vi "Configure Steering Frame.vi"(8 "error in (no error)":errorcluster, 10 "dialog options in":variant, 11 "steering frame in":refnum<class "NI_Robotics_Steering Frame.lvclass">) -> (0 "error out":errorcluster, 1 "cancelled?":bool, 2 "dialog options out":variant, 3 "steering frame out":refnum<class "NI_Robotics_Steering Frame.lvclass">, 5 "steering type":string)   [LabVIEW 2017, in "NI_Robotics_Configure Steering Frame.lvlib"]
uses:
  <vilib>/robotics/Dialog/Configure Steering Frame/NI_Robotics_Configure Steering Frame.lvlib
  <vilib>/robotics/Dialog/Configure Steering Frame/Steering Type.ctl
  <vilib>/robotics/Dialog/Configure Steering Frame/Zoom Extent.ctl
  <vilib>/robotics/Dialog/Configure Steering Frame/Zoom In.ctl
  <vilib>/robotics/Dialog/Configure Steering Frame/Zoom Out.ctl
  <vilib>/robotics/Dialog/Configure Steering Frame/Copy.ctl
  <vilib>/robotics/Dialog/Configure Steering Frame/Remove.ctl
  <vilib>/robotics/Dialog/Configure Steering Frame/Add.ctl
  <vilib>/robotics/Dialog/Configure Steering Frame/Angle Mode.ctl
  <vilib>/robotics/Steering/Steering Frame/NI_Robotics_Steering Frame.lvclass
  <vilib>/robotics/Dialog/Configure Steering Frame/FP Refs.ctl
  <vilib>/Utility/cursorutil.llb/Set Cursor (Icon Pict).vi
  <vilib>/robotics/Dialog/Configure Steering Frame/Global Strings.vi
panel:
  in  "Angle Units":T1=1 items=["Degrees", "Radians"]
  in  "help":bool
  in  "cancel":bool
  in  "ok":bool
  in  "Copy Wheel":T2
  in  "Remove Wheel":T3
  in  "Add Wheel":T4
  in  "Wheels":i32[](listbox)=[0]
  in  "zoom extent":T5 caption="Zoom to Fit"
  in  "zoom out":T6 caption="Zoom Out"
  in  "zoom in":T7 caption="Zoom In"
  in  "Steering Type":T8 items=["User Defined", "Differential", "Ackermann", "Mecanum"]
  out "picture":picture
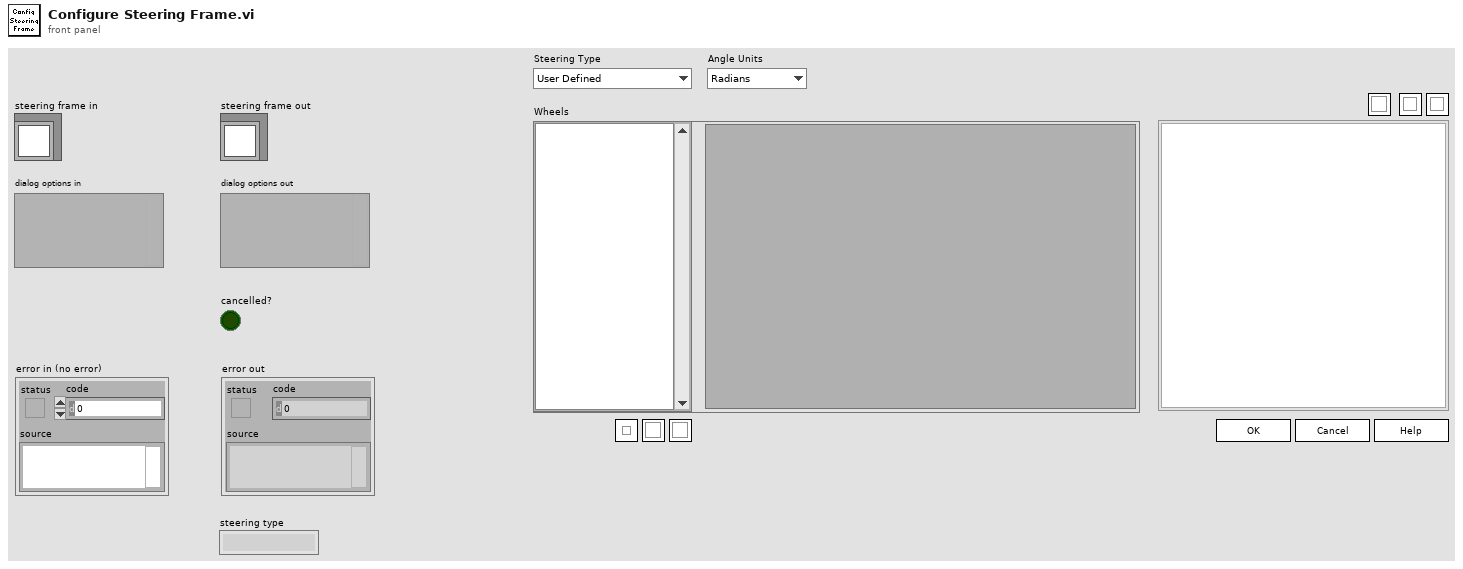
[diagram p1: front panel]
types:
  T1 = typedef "NI_Robotics_Configure Steering Frame.lvlib/Angle Mode.ctl" = u16
  T2 = typedef "NI_Robotics_Configure Steering Frame.lvlib/Copy.ctl" = bool
  T3 = typedef "NI_Robotics_Configure Steering Frame.lvlib/Remove.ctl" = bool
  T4 = typedef "NI_Robotics_Configure Steering Frame.lvlib/Add.ctl" = bool
  T5 = typedef "NI_Robotics_Configure Steering Frame.lvlib/Zoom Extent.ctl" = bool
  T6 = typedef "NI_Robotics_Configure Steering Frame.lvlib/Zoom Out.ctl" = bool
  T7 = typedef "NI_Robotics_Configure Steering Frame.lvlib/Zoom In.ctl" = bool
  T8 = typedef "NI_Robotics_Configure Steering Frame.lvlib/Steering Type.ctl" = u16
  T9 = typedef "NI_Robotics_Configure Steering Frame.lvlib/FP Refs.ctl" = cluster{"VI Refnum":refnum<vi>, "Menu Ref":refnum<k9>, "Sub Panel":refnum<vi>, "picture":refnum<vi>, "Steering Type":refnum<vi>, "zoom in":refnum<vi>, "zoom out":refnum<vi>, "zoom extents":refnum<vi>, "Wheels":refnum<vi>, "Add Wheel":refnum<vi>, "Remove Wheel":refnum<vi>, "Copy Wheel":refnum<vi>, "Angle Units":refnum<vi>}
  T10 = typedef "NI_Robotics_Configure Steering Frame.lvlib/Dialog Options.ctl" = cluster{"angle mode":T1, "picture pixels per unit":dbl, "close window on exit":bool, "window behavior":enum32{"Invalid", "Default", "Floating", "Floating/Auto-Hide", "Modal"}}
  T11 = typedef "NI_Robotics_Configure Steering Frame.lvlib/Subpanel to Main Command Event Reg.ctl" = refnum<event-registration>
  T12 = typedef "NI_Robotics_Configure Steering Frame.lvlib/Dialog Info.ctl" = cluster{"steering frame ref":refnum<data-value>, "active wheel indexes":i32[], "FP Refs":T9, "subpanel info":T13, "picture dragging state":T15, "picture size (pixels)":T17, "picture grid":picture, "click zones group":cluster{"click zones array":T18[], "num click zones":i32}, "draw options":T19}
  T13 = typedef "NI_Robotics_Configure Steering Frame.lvlib/Subpanel Info.ctl" = cluster{"subpanel VI refs":refnum<vi>[], "subpanel types":string[], "main to subpanel command events":T14[]}
  T14 = typedef "NI_Robotics_Configure Steering Frame.lvlib/Main to Subpanel Command Event.ctl" = refnum<user-event>
  T15 = typedef "NI_Robotics_Configure Steering Frame.lvlib/Dragging State.ctl" = cluster{"dragging":bool, "wheel index":i32, "dragging mode":T16, "wheel start position":cluster{"x":dbl, "y":dbl, "theta":dbl}, "relative mouse position":cluster{"x":dbl, "y":dbl}, "relative mouse init angle (rad)":dbl}
  T16 = typedef "NI_Robotics_Configure Steering Frame.lvlib/Dragging Mode.ctl" = enum16{"translate", "rotate"}
  T17 = typedef "LVBoundsTypeDef.ctl" = cluster{"Width":u32, "Height":u32}
  T18 = typedef "NI_Robotics_Configure Steering Frame.lvlib/Click Zone.ctl" = cluster{"wheel index":i32, "global coordinate":cluster{"x":dbl, "y":dbl}, "radius":dbl}
  T19 = typedef "NI_Robotics_Steering Picture.lvlib/Draw Steering Frame Options.ctl" = cluster{"draw wheel states?":bool, "highlight wheel index":i32, "pixels per unit":dbl, "draw forward velocity?":bool, "velocity scale":dbl}
  T20 = typedef "eventvkey.ctl" = enum16{"ASCII", "Enter", "Return", "Shift", "Ctrl", "Alt", "Cmd", "Opt", "Caps", "NumLock", "Clear", "Break", "Up", "Down", "Left", "Right", "Insert", "Delete", "Home", "End", "PageUp", "PageDown", "Escape", "Help", "Pause", "ScrollLock", "F1", "F2", "F3", "F4", "F5", "F6", "F7", "F8", "F9", "F10", "F11", "F12", "F13", "F14", "F15", "F16", "F17", "F18", "F19", "F20", "F21", "F22", "F23", "F24", "Play", "VolumeUp", "VolumeDown", "Mute", "Two Byte Char"}
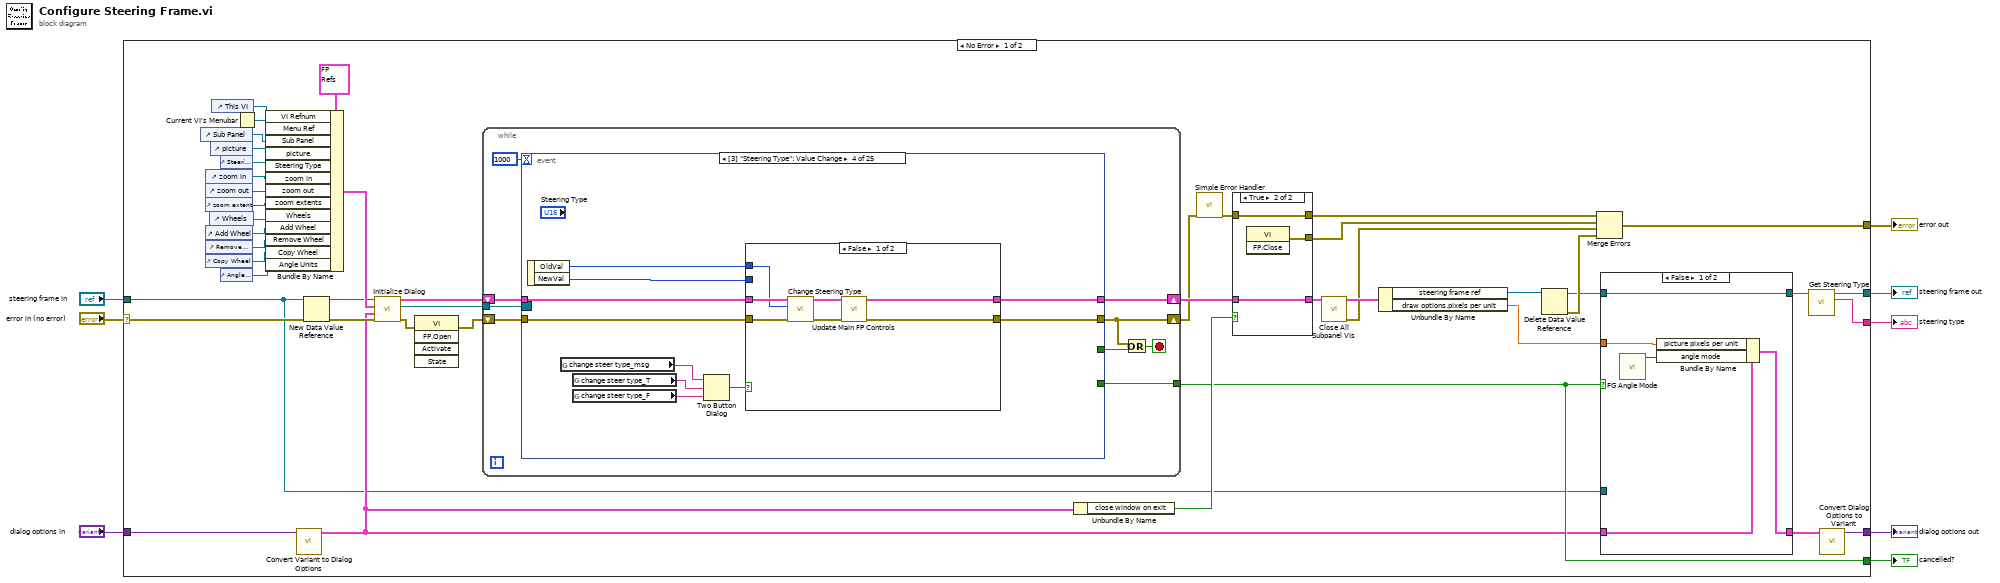
[diagram p0: block diagram]
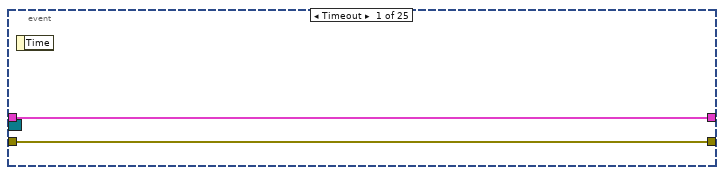
[diagram p4: hidden frame]
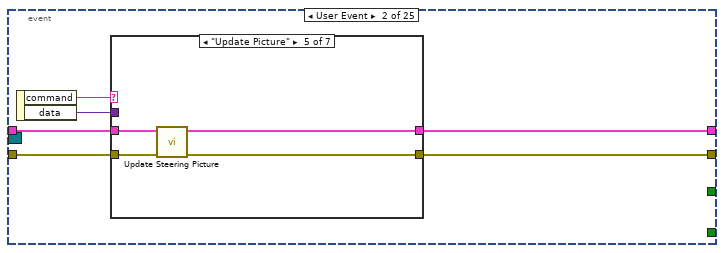
[diagram p5: hidden frame]
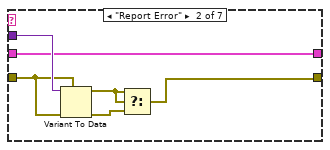
[diagram p7: hidden frame]
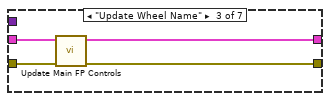
[diagram p8: hidden frame]
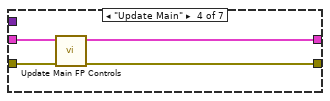
[diagram p9: hidden frame]
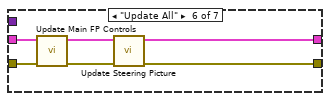
[diagram p10: hidden frame]
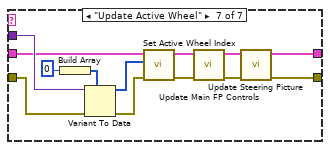
[diagram p11: hidden frame]
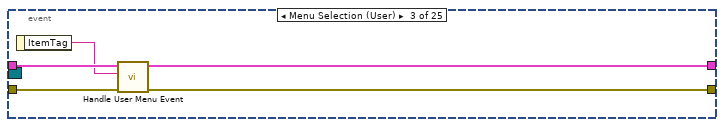
[diagram p12: hidden frame]
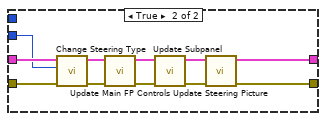
[diagram p13: hidden frame]
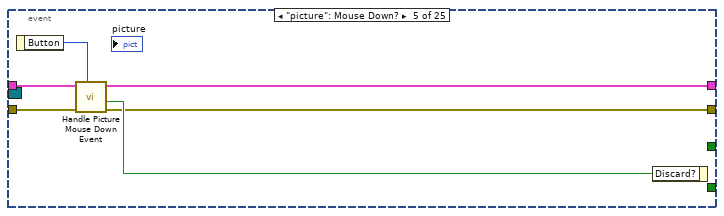
[diagram p14: hidden frame]
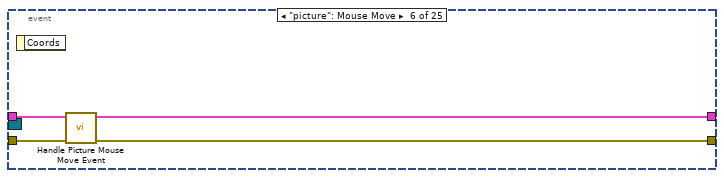
[diagram p15: hidden frame]
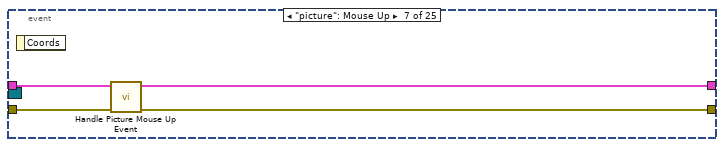
[diagram p16: hidden frame]
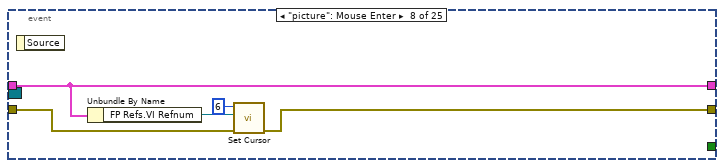
[diagram p17: hidden frame]
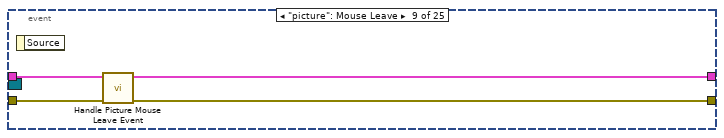
[diagram p18: hidden frame]
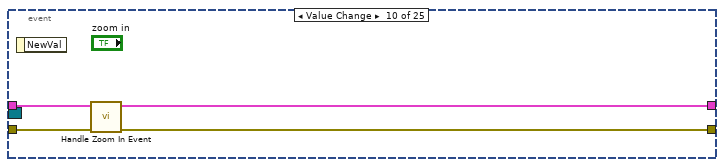
[diagram p19: hidden frame]
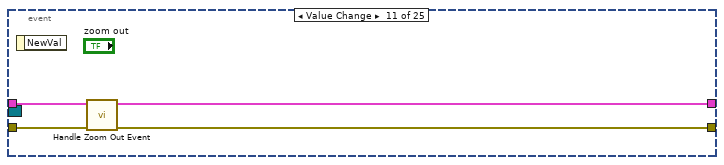
[diagram p20: hidden frame]
diagram:
  n1 = case shown="No Error" "error in (no error)" {
    selector: "error in (no error)" -> [w25 w319]
    tunnel: [w15 w317] -> w1
    tunnel: [w32 _] -> w8
    tunnel: "dialog options in" -> [w21 w318]
    tunnel: [w19 w318] -> w6
    tunnel: [w30 w319] -> w3
    tunnel: [w16 _] -> w4
    tunnel: "steering frame in" -> [w9 w317]
    frame No Error {
      n2 = control-ref of="Sub Panel"() -> (w52:refnum<vi>)
      n3 = control-ref of="zoom in"() -> (w29:refnum<vi>)
      n4 = control-ref of="zoom out"() -> (w28:refnum<vi>)
      n5 = control-ref of="zoom extent"() -> (w27:refnum<vi>)
      n6 = control-ref of="Add Wheel"() -> (w24:refnum<vi>)
      n7 = control-ref of="Remove Wheel"() -> (w23:refnum<vi>)
      n8 = control-ref of="Copy Wheel"() -> (w22:refnum<vi>)
      n9 = control-ref of="Wheels"() -> (w14:refnum<vi>)
      n10 = control-ref of="picture"() -> (w48:refnum<vi>)
      n11 = control-ref of="This VI"() -> (w46:refnum<vi>)
      n12 = control-ref of="Steering Type"() -> (w11:refnum<vi>)
      n13 = control-ref of="Angle Units"() -> (w10:refnum<vi>)
      n14 = Current VI's Menubar() -> (w31:refnum<k9>)
      n15 = Bundle By Name(cluster=T9 {"VI Refnum"=refnum, "Menu Ref"=refnum, "Sub Panel"=refnum, "picture"=refnum, "Steering Type"=refnum, "zoom in"=refnum, "zoom out"=refnum, "zoom extents"=refnum, "Wheels"=refnum, "Add Wheel"=refnum, "Remove Wheel"=refnum, "Copy Wheel"=refnum, "Angle Units"=refnum} ("FP Refs"), "VI Refnum"=w46, "Menu Ref"=w31, "Sub Panel"=w52, "picture"=w48, "Steering Type"=w11, "zoom in"=w29, "zoom out"=w28, "zoom extents"=w27, "Wheels"=w14, "Add Wheel"=w24, "Remove Wheel"=w23, "Copy Wheel"=w22, "Angle Units"=w10) -> (w49:T9)
      n16 = call <vilib>:"Convert Variant to Dialog Options.vi"("dialog options variant"=w21) -> ("dialog options"=w20:T10)  [unwired: 9 in, 1 out]
      n17 = New Data Value Reference(data value=w9, error in=w25) -> (data value reference=w43:refnum<data-value>, error out=w42:errorcluster)
      n18 = call <vilib>:"Initialize Dialog.vi"("error in (no error)"=w42, "dialog options in"=w20, "FP Refs"=w49, "steering frame ref in"=w43) -> ("error out"=w45:errorcluster, "subpanel to main command event reg"=w51:T11, "dialog info"=w50:T12)  [unwired: 5 in]
      n19 = invoke class="VI" method="FP.Open"(error in=w45) -> (error out=w44:errorcluster)  [unwired: 4 in, 4 out]
      n20 = while {
        shift-right: [w66] -> w13
        shift-left: w44 -> [w73]
        tunnel: w51 -> [w74]
        shift-right: [w68] -> w40
        shift-left: w50 -> [w71]
        tunnel: [w67] -> w32
        stop <- w70 stop-if-true
        n21 = event shown="[3] \"Steering Type\": Value Change" {
          selector: w74 -> [_ _ _ _ _ _ _ _ _ _ _ _ _ _ _ _ _ _ _ _ _ _ _ _ _]
          dyn-events: _ -> [_ _ _ _ _ _ _ _ _ _ _ _ _ _ _ _ _ _ _ _ _ _ _ _ _]
          timeout: 1000 -> [_ _ _ _ _ _ _ _ _ _ _ _ _ _ _ _ _ _ _ _ _ _ _ _ _]
          tunnel: w73 -> [w76 w80 w124 w135 w156 w163 w166 w170 w175 w179 w183 w190 w194 w198 w207 w231 w236 w241 w266 w282 w296 w300 w304 w306 w316]
          tunnel: [w76 w79 w123 w134 w158 w161 w165 w169 w174 w178 w182 w187 w193 w202 w206 w230 w235 w248 w262 w278 w290 w300 w304 w305 w316] -> w66
          tunnel: [w75 w77 w125 w132 w159 w162 w167 w171 w176 w180 w184 w188 w195 w204 w208 w232 w237 w249 w263 w279 w293 w301 w303 w309 w315] -> w68
          tunnel: w71 -> [w75 w78 w126 w133 w157 w164 w168 w171 w177 w181 w185 w189 w196 w201 w209 w233 w238 w243 w267 w283 w294 w301 w303 w309 w315]
          tunnel: [_ _ _ _ _ _ _ _ _ _ _ _ _ _ _ _ _ _ _ _ _ TRUE w302 _ w310] -> w69
          tunnel: [_ _ _ _ _ _ _ _ _ _ _ _ _ _ _ _ _ _ _ _ _ _ w302 _ w310] -> w67
          event Timeout {
            n22 = event-data() -> ()  [unwired: 1 in, 1 out]
          }
          event User Event {
            n23 = event-data() -> ("command"=w82:string, "data"=w81:variant)  [unwired: 1 in]
            n24 = case shown="\"Update Picture\"" w82 {
              tunnel: w81 -> [_ w90 _ _ _ _ w121]
              tunnel: w80 -> [w84 w89 w92 w96 w101 w107 w120]
              tunnel: [w84 w86 w91 w95 w99 w103 w116] -> w79
              tunnel: w78 -> [w83 w85 w94 w98 w102 w108 w115]
              tunnel: [w83 w85 w93 w97 w100 w104 w117] -> w77
              frame Default {
              }
              frame "Report Error" {
                n25 = Variant To Data(error in=w89, type=w89, Variant=w90) -> (data=w88:errorcluster, error out=w87:errorcluster)
                n26 = Select(t=w88, s=w88, f=w87) -> (s? t:f=w86:errorcluster)
              }
              frame "Update Wheel Name" {
                n27 = call <vilib>:"Update Main FP Controls.vi"("error in (no error)"=w92, "dialog info in"=w94) -> ("error out"=w91:errorcluster, "dialog info out"=w93:T12)  [unwired: 8 in]
              }
              frame "Update Main" {
                n28 = call <vilib>:"Update Main FP Controls.vi"("error in (no error)"=w96, "dialog info in"=w98) -> ("error out"=w95:errorcluster, "dialog info out"=w97:T12)  [unwired: 8 in]
              }
              frame "Update Picture" {
                n29 = call <vilib>:"Update Steering Picture.vi"("error in (no error)"=w101, "dialog info in"=w102) -> ("error out"=w99:errorcluster, "dialog info out"=w100:T12)  [unwired: 8 in]
              }
              frame "Update All" {
                n30 = call <vilib>:"Update Main FP Controls.vi"("error in (no error)"=w107, "dialog info in"=w108) -> ("error out"=w105:errorcluster, "dialog info out"=w106:T12)  [unwired: 8 in]
                n31 = call <vilib>:"Update Steering Picture.vi"("error in (no error)"=w105, "dialog info in"=w106) -> ("error out"=w103:errorcluster, "dialog info out"=w104:T12)  [unwired: 8 in]
              }
              frame "Update Active Wheel" {
                n32 = Build Array(0) -> (w109:i32[])
                n33 = Variant To Data(error in=w120, type=w109, Variant=w121) -> (data=w114:i32[], error out=w113:errorcluster)
                n34 = call <vilib>:"Set Active Wheel Index.vi"("error in (no error)"=w113, "active wheel indexes"=w114, "dialog info in"=w115) -> ("error out"=w112:errorcluster, "dialog info out"=w111:T12)  [unwired: 7 in]
                n35 = call <vilib>:"Update Main FP Controls.vi"("error in (no error)"=w112, "dialog info in"=w111) -> ("error out"=w118:errorcluster, "dialog info out"=w119:T12)  [unwired: 8 in]
                n36 = call <vilib>:"Update Steering Picture.vi"("error in (no error)"=w118, "dialog info in"=w119) -> ("error out"=w116:errorcluster, "dialog info out"=w117:T12)  [unwired: 8 in]
              }
            }
          }
          event Menu Selection (User) {
            n37 = event-data() -> ("ItemTag"=w122:string)  [unwired: 1 in]
            n38 = call <vilib>:"Handle User Menu Event.vi"("error in (no error)"=w124, "item tag"=w122, "dialog info in"=w126) -> ("error out"=w123:errorcluster, "dialog info out"=w125:T12)  [unwired: 7 in]
          }
          event Value Change {
            n39 = event-data() -> ("OldVal"=w130:T8, "NewVal"=w131:T8)  [unwired: 1 in]
            n40 = global read "Global Strings.vi" "change steer type_msg"() -> (w129:string)
            n41 = global read "Global Strings.vi" "change steer type_T"() -> (w128:string)
            n42 = global read "Global Strings.vi" "change steer type_F"() -> (w127:string)
            n43 = Two Button Dialog(message=w129, 1:w127, 2:w128) -> (T button?=w136:bool)
            n44 = case shown="False" w136 {
              tunnel: w135 -> [w142 w153]
              tunnel: [w137 w148] -> w134
              tunnel: w133 -> [w143 w154]
              tunnel: [w139 w150] -> w132
              tunnel: w131 -> [_ w152]
              tunnel: w130 -> [w141 _]
              frame False {
                n45 = call <vilib>:"Change Steering Type.vi"("error in (no error)"=w142, "steering type"=w141, "dialog info in"=w143) -> ("error out"=w138:errorcluster, "dialog info out"=w140:T12)  [unwired: 7 in]
                n46 = call <vilib>:"Update Main FP Controls.vi"("error in (no error)"=w138, "dialog info in"=w140) -> ("error out"=w137:errorcluster, "dialog info out"=w139:T12)  [unwired: 8 in]
              }
              frame True {
                n47 = call <vilib>:"Change Steering Type.vi"("error in (no error)"=w153, "steering type"=w152, "dialog info in"=w154) -> ("error out"=w145:errorcluster, "dialog info out"=w147:T12)  [unwired: 7 in]
                n48 = call <vilib>:"Update Main FP Controls.vi"("error in (no error)"=w145, "dialog info in"=w147) -> ("error out"=w144:errorcluster, "dialog info out"=w146:T12)  [unwired: 8 in]
                n49 = call <vilib>:"Update Subpanel.vi"("error in (no error)"=w144, "dialog info in"=w146) -> ("error out"=w149:errorcluster, "dialog info out"=w151:T12)  [unwired: 8 in]
                n50 = call <vilib>:"Update Steering Picture.vi"("error in (no error)"=w149, "dialog info in"=w151) -> ("error out"=w148:errorcluster, "dialog info out"=w150:T12)  [unwired: 8 in]
              }
            }
          }
          event "picture": Mouse Down? {
            n51 = event-data() -> ("Button"=w155:u16)  [unwired: 1 in]
            n52 = call <vilib>:"Handle Picture Mouse Down Event.vi"("Button"=w155, "error in (no error)"=w156, "dialog info in"=w157) -> ("error out"=w158:errorcluster, "discard?"=w160:bool, "dialog info out"=w159:T12)  [unwired: 6 in]
            n53 = event-data("Discard?"=w160) -> ()  [unwired: 1 in, 1 out]
          }
          event "picture": Mouse Move {
            n54 = event-data() -> ()  [unwired: 1 in, 1 out]
            n55 = call <vilib>:"Handle Picture Mouse Move Event.vi"("error in (no error)"=w163, "dialog info in"=w164) -> ("error out"=w161:errorcluster, "dialog info out"=w162:T12)  [unwired: 8 in]
          }
          event "picture": Mouse Up {
            n56 = event-data() -> ()  [unwired: 1 in, 1 out]
            n57 = call <vilib>:"Handle Picture Mouse Up Event.vi"("error in (no error)"=w166, "dialog info in"=w168) -> ("error out"=w165:errorcluster, "dialog info out"=w167:T12)  [unwired: 8 in]
          }
          event "picture": Mouse Enter {
            n58 = event-data() -> ()  [unwired: 1 in, 1 out]
            n59 = Unbundle By Name(w171) -> ("FP Refs.VI Refnum"=w172:refnum<vi>)
            n60 = call-poly <vilib>:"Set Cursor.vi"("error in (no error)"=w170, "VI reference (current VI)"=w172, "icon"=u16 6) -> ("error out"=w169:errorcluster)  [unwired: 7 in, 1 out]
          }
          event "picture": Mouse Leave {
            n61 = event-data() -> ()  [unwired: 1 in, 1 out]
            n62 = call <vilib>:"Handle Picture Mouse Leave Event.vi"("error in (no error)"=w175, "dialog info in"=w177) -> ("error out"=w174:errorcluster, "dialog info out"=w176:T12)  [unwired: 8 in]
          }
          event Value Change {
            n63 = event-data() -> ()  [unwired: 1 in, 1 out]
            n64 = call <vilib>:"Handle Zoom In Event.vi"("error in (no error)"=w179, "dialog info in"=w181) -> ("error out"=w178:errorcluster, "dialog info out"=w180:T12)  [unwired: 8 in]
          }
          event Value Change {
            n65 = event-data() -> ()  [unwired: 1 in, 1 out]
            n66 = call <vilib>:"Handle Zoom Out Event.vi"("error in (no error)"=w183, "dialog info in"=w185) -> ("error out"=w182:errorcluster, "dialog info out"=w184:T12)  [unwired: 8 in]
          }
          event Value Change {
            w186 = TRUE ("zoom to fit (F)")
            n67 = event-data() -> ()  [unwired: 1 in, 1 out]
            n68 = call <vilib>:"Update Steering Picture.vi"("redraw grid (F)"=w186, "zoom to fit (F)"=w186, "error in (no error)"=w190, "dialog info in"=w189) -> ("error out"=w187:errorcluster, "dialog info out"=w188:T12)  [unwired: 6 in]
          }
          event "picture": Key Down? {
            n69 = event-data() -> ("VKey"=w192:T20)  [unwired: 1 in]
            n70 = call <vilib>:"Handle Picture Key Down Event.vi"("VKey"=w192, "error in (no error)"=w194, "dialog info in"=w196) -> ("error out"=w193:errorcluster, "discard?"=w191:bool, "dialog info out"=w195:T12)  [unwired: 6 in]
            n71 = event-data("Discard?"=w191) -> ()  [unwired: 1 in, 1 out]
          }
          event "Wheels": Value Change {
            n72 = event-data() -> ("NewVal"=w199:i32[])  [unwired: 1 in]
            n73 = call <vilib>:"Set Active Wheel Index.vi"("error in (no error)"=w198, "active wheel indexes"=w199, "dialog info in"=w201) -> ("error out"=w197:errorcluster, "dialog info out"=w200:T12)  [unwired: 7 in]
            n74 = call <vilib>:"Update Steering Picture.vi"("error in (no error)"=w197, "dialog info in"=w200) -> ("error out"=w203:errorcluster, "dialog info out"=w205:T12)  [unwired: 8 in]
            n75 = call <vilib>:"Update Subpanel.vi"("error in (no error)"=w203, "dialog info in"=w205) -> ("error out"=w202:errorcluster, "dialog info out"=w204:T12)  [unwired: 8 in]
          }
          event "Wheels": Key Down? {
            n76 = event-data() -> ("VKey"=w210:T20)  [unwired: 1 in]
            n77 = case shown="\"Delete\"" w210 {
              tunnel: w209 -> [w212 w222]
              tunnel: [w212 w221] -> w208
              tunnel: w207 -> [w211 w219]
              tunnel: [w211 w220] -> w206
              frame Default {
              }
              frame "Delete" {
                n78 = in-place {
                  in-place-border: w219 -> [w224]
                  in-place-border: [w223] -> w214
                  n79 = in-place-cluster #1(w222) -> ("steering frame ref"=w228:refnum<data-value>, "active wheel indexes"=w227:i32[])
                  n80 = call <vilib>:"Remove Wheel.vi"("error in (no error)"=w224, "active wheel indexes in"=w227, "steering frame ref in"=w228) -> ("error out"=w223:errorcluster, "active wheel indexes out"=w226:i32[], "steering frame ref out"=w225:refnum<data-value>)  [unwired: 5 in, 1 out]
                  n81 = in-place-cluster #1("steering frame ref"=w225, "active wheel indexes"=w226) -> (w216:T12)
                }
                n82 = call <vilib>:"Update Main FP Controls.vi"("error in (no error)"=w214, "dialog info in"=w216) -> ("error out"=w213:errorcluster, "dialog info out"=w215:T12)  [unwired: 8 in]
                n83 = call <vilib>:"Update Steering Picture.vi"("error in (no error)"=w213, "dialog info in"=w215) -> ("error out"=w217:errorcluster, "dialog info out"=w218:T12)  [unwired: 8 in]
                n84 = call <vilib>:"Update Subpanel.vi"("error in (no error)"=w217, "dialog info in"=w218) -> ("error out"=w220:errorcluster, "dialog info out"=w221:T12)  [unwired: 8 in]
              }
            }
            n85 = event-data() -> ()  [unwired: 2 in, 1 out]
          }
          event "Wheels": Shortcut Menu Activation? {
            n86 = event-data() -> ("MenuRef"=w229:refnum<k9>)  [unwired: 1 in]
            n87 = call <vilib>:"Handle Listbox Shortcut Activation Event.vi"("error in (no error)"=w231, "MenuRef"=w229, "dialog info in"=w233) -> ("error out"=w230:errorcluster, "dialog info out"=w232:T12)  [unwired: 7 in]
            n88 = event-data() -> ()  [unwired: 2 in, 1 out]
          }
          event "Wheels": Shortcut Menu Selection (User) {
            n89 = event-data() -> ("ItemTag"=w234:string)  [unwired: 1 in]
            n90 = call <vilib>:"Handle Listbox Shortcut Selection Event.vi"("error in (no error)"=w236, "Item Tag"=w234, "dialog info in"=w238) -> ("error out"=w235:errorcluster, "dialog info out"=w237:T12)  [unwired: 7 in]
          }
          event Value Change {
            n91 = event-data() -> ()  [unwired: 1 in, 1 out]
            n92 = call <vilib>:"Generate Unique Wheel Name.vi"("error in (no error)"=w241, "dialog info in"=w243) -> ("error out"=w240:errorcluster, "unique name"=w239:string, "dialog info out"=w242:T12)  [unwired: 7 in]
            n93 = in-place {
              in-place-border: w240 -> [w254]
              in-place-border: [w253] -> w245
              in-place-border: w239 -> [w252]
              n94 = in-place-cluster #2(w242) -> ("steering frame ref"=w257:refnum<data-value>)  [unwired: 1 out]
              n95 = call <vilib>:"Add Fixed Wheel.vi"("error in (no error)"=w254, "wheel name"=w252, "steering frame ref in"=w257) -> ("error out"=w253:errorcluster, "active wheel indexes out"=w255:i32[], "steering frame ref out"=w256:refnum<data-value>)  [unwired: 6 in]
              n96 = in-place-cluster #2("steering frame ref"=w256, "active wheel indexes"=w255) -> (w247:T12)
            }
            n97 = call <vilib>:"Update Main FP Controls.vi"("error in (no error)"=w245, "dialog info in"=w247) -> ("error out"=w244:errorcluster, "dialog info out"=w246:T12)  [unwired: 8 in]
            n98 = call <vilib>:"Update Steering Picture.vi"("error in (no error)"=w244, "dialog info in"=w246) -> ("error out"=w250:errorcluster, "dialog info out"=w251:T12)  [unwired: 8 in]
            n99 = call <vilib>:"Update Subpanel.vi"("error in (no error)"=w250, "dialog info in"=w251) -> ("error out"=w248:errorcluster, "dialog info out"=w249:T12)  [unwired: 8 in]
          }
          event Value Change {
            n100 = event-data() -> ()  [unwired: 1 in, 1 out]
            n101 = in-place {
              in-place-border: w266 -> [w269]
              in-place-border: [w268] -> w259
              n102 = in-place-cluster #3(w267) -> ("steering frame ref"=w273:refnum<data-value>, "active wheel indexes"=w271:i32[])
              n103 = call <vilib>:"Remove Wheel.vi"("error in (no error)"=w269, "active wheel indexes in"=w271, "steering frame ref in"=w273) -> ("error out"=w268:errorcluster, "active wheel indexes out"=w270:i32[], "steering frame ref out"=w272:refnum<data-value>)  [unwired: 5 in, 1 out]
              n104 = in-place-cluster #3("steering frame ref"=w272, "active wheel indexes"=w270) -> (w261:T12)
            }
            n105 = call <vilib>:"Update Main FP Controls.vi"("error in (no error)"=w259, "dialog info in"=w261) -> ("error out"=w258:errorcluster, "dialog info out"=w260:T12)  [unwired: 8 in]
            n106 = call <vilib>:"Update Steering Picture.vi"("error in (no error)"=w258, "dialog info in"=w260) -> ("error out"=w264:errorcluster, "dialog info out"=w265:T12)  [unwired: 8 in]
            n107 = call <vilib>:"Update Subpanel.vi"("error in (no error)"=w264, "dialog info in"=w265) -> ("error out"=w262:errorcluster, "dialog info out"=w263:T12)  [unwired: 8 in]
          }
          event Value Change {
            n108 = event-data() -> ()  [unwired: 1 in, 1 out]
            n109 = in-place {
              in-place-border: w282 -> [w285]
              in-place-border: [w284] -> w275
              n110 = in-place-cluster #4(w283) -> ("steering frame ref"=w289:refnum<data-value>, "active wheel indexes"=w287:i32[])
              n111 = call <vilib>:"Copy Wheel.vi"("error in (no error)"=w285, "active wheel indexes in"=w287, "steering frame ref in"=w289) -> ("error out"=w284:errorcluster, "active wheel indexes out"=w286:i32[], "steering frame ref out"=w288:refnum<data-value>)  [unwired: 5 in, 1 out]
              n112 = in-place-cluster #4("steering frame ref"=w288, "active wheel indexes"=w286) -> (w277:T12)
            }
            n113 = call <vilib>:"Update Main FP Controls.vi"("error in (no error)"=w275, "dialog info in"=w277) -> ("error out"=w274:errorcluster, "dialog info out"=w276:T12)  [unwired: 8 in]
            n114 = call <vilib>:"Update Steering Picture.vi"("error in (no error)"=w274, "dialog info in"=w276) -> ("error out"=w280:errorcluster, "dialog info out"=w281:T12)  [unwired: 8 in]
            n115 = call <vilib>:"Update Subpanel.vi"("error in (no error)"=w280, "dialog info in"=w281) -> ("error out"=w278:errorcluster, "dialog info out"=w279:T12)  [unwired: 8 in]
          }
          event Value Change {
            n116 = event-data() -> ("NewVal"=w297:T1)  [unwired: 1 in]
            n117 = call <vilib>:"FG Angle Mode.vi"("action (read)"=enum16{"read", "write"}."write", "error in (no error)"=w296, "angle mode in"=w297) -> ("error out"=w291:errorcluster)  [unwired: 7 in, 1 out]
            n118 = call <vilib>:"Update Subpanel.vi"("error in (no error)"=w291, "dialog info in"=w294) -> ("error out"=w292:errorcluster, "dialog info out"=w295:T12)  [unwired: 8 in]
            n119 = call <vilib>:"Update Main FP Controls.vi"("error in (no error)"=w292, "dialog info in"=w295) -> ("error out"=w290:errorcluster, "dialog info out"=w293:T12)  [unwired: 8 in]
          }
          event "ok": Value Change {
            n120 = event-data() -> ()  [unwired: 1 in, 1 out]
          }
          event "cancel": Value Change {
            w302 = TRUE
            n121 = event-data() -> ()  [unwired: 1 in, 1 out]
          }
          event "help": Value Change {
            n122 = event-data() -> ()  [unwired: 1 in, 1 out]
            n123 = call <helpdir>:"_LaunchHelp.vi"("error in (no error)"=w306, "CHM or HLP filename (lvdialog.chm)"="lvrobovi.chm", "HTML filename"="config_steering_frame.html") -> ("error out"=w305:errorcluster)  [unwired: 4 out]
          }
          event Panel Close? {
            n124 = event-data() -> ()  [unwired: 1 in, 1 out]
            n125 = Two Button Dialog(message="Are you sure you want to cancel?", 1:"No" ("F button name (\"Cancel\")"), 2:"Yes" ("T button name (\"OK\")")) -> (T button?=w310:bool)
            n126 = event-data("Discard?"=TRUE) -> ()  [unwired: 1 in, 1 out]
          }
        }
        n127 = Or(x=w66, y=w69) -> (x .or. y?=w70:bool)
      }
      n128 = Unbundle By Name(w20) -> ("close window on exit"=w33:bool)
      n129 = call <vilib>:"Simple Error Handler.vi"("error in (no error)"=w13) -> ("error out"=w12:errorcluster)  [unwired: 4 in, 4 out]
      n130 = case shown="True" w33 {
        tunnel: w12 -> [w62 w64]
        tunnel: w40 -> [w61 w65]
        tunnel: [w61 w65] -> w39
        tunnel: [w62 w64] -> w38
        tunnel: [_ w63] -> w37
        frame False {
        }
        frame True {
          n131 = invoke class="VI" method="FP.Close"() -> (error out=w63:errorcluster)  [unwired: 3 in, 2 out]
        }
      }
      n132 = call <vilib>:"Close All Subpanel VIs.vi"("dialog info in"=w39) -> ("error out"=w36:errorcluster, "dialog info out"=w47:T12)  [unwired: 9 in]
      n133 = Unbundle By Name(w47) -> ("steering frame ref"=w41:refnum<data-value>, "draw options.pixels per unit"=w26:dbl)
      n134 = Delete Data Value Reference(data value reference=w41) -> (data value=w34:refnum<class "NI_Robotics_Steering Frame.lvclass">, error out=w35:errorcluster)  [unwired: 1 in]
      n135 = Merge Errors(w38, w37, w36, w35) -> (w30:errorcluster)
      n136 = case shown="False" w32 {
        tunnel: w34 -> [w58 _]
        tunnel: [w58 w60] -> w17
        tunnel: w9 -> [_ w60]
        tunnel: w20 -> [w56 w59]
        tunnel: [w55 w59] -> w18
        tunnel: w26 -> [w54 _]
        frame False {
          n137 = call <vilib>:"FG Angle Mode.vi"() -> ("angle mode out"=w57:T1)  [unwired: 10 in, 1 out]
          n138 = Bundle By Name(cluster=w56, "picture pixels per unit"=w54, "angle mode"=w57) -> (w55:T10)
        }
        frame True {
        }
      }
      n139 = call-dynamic "Get Steering Type.vi"("steering frame in"=w17) -> ("steering type"=w16:string, "steering frame out"=w15:refnum<class "NI_Robotics_Steering Frame.lvclass">)  [unwired: 8 in, 1 out]
      n140 = call <vilib>:"Convert Dialog Options to Variant.vi"("dialog options"=w18) -> ("dialog options variant"=w19:variant)  [unwired: 9 in, 1 out]
    }
    frame Error {
    }
  }
  "error out" <- w3
  "cancelled?" <- w8
  "dialog options out" <- w6
  "steering type" <- w4
  "steering frame out" <- w1
